vi "RenameMembersSetName.vi"(4 "Output String":string, 6 "Input String":string, 8 "error in (no error)":errorcluster, 10 "Controls":refnum<vi>[](array[refnum]), 11 "LVClassLibrary Refnum":refnum<vi>) -> (0 "error out":errorcluster, 3 "Library Refnum out":refnum<vi>)   [LabVIEW 2014, in "ClassRenamer.lvclass"]
uses:
  ClassRenamer.lvclass
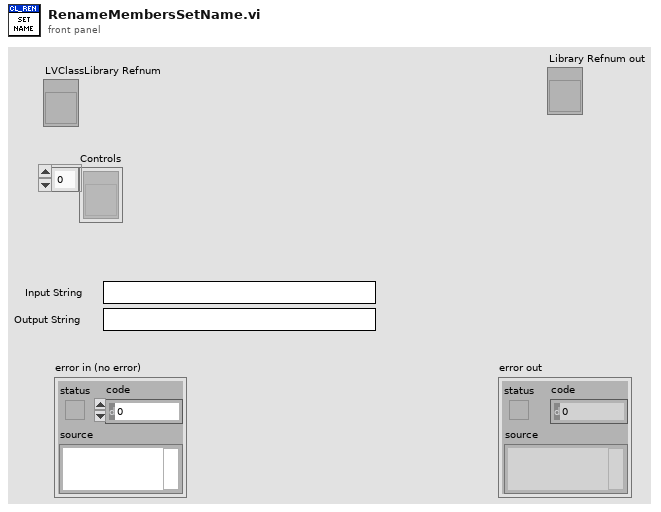
[diagram p1: front panel]
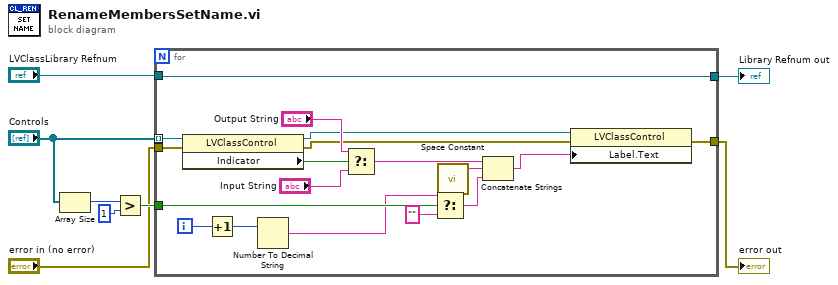
[diagram p0: block diagram]
diagram:
  n1 = Array Size(array="Controls") -> (size(s)=w7:i32)
  n2 = Greater?(x=w7, y=1) -> (0:w4:bool)
  n3 = for {
    tunnel: "Controls" -> [w23] mode=indexing
    tunnel: "LVClassLibrary Refnum" -> [w19]
    tunnel: w4 -> [w16]
    tunnel: [w19] -> w3
    tunnel: "error in (no error)" -> [w18]
    tunnel: [w9] -> w1
    i -> [w26]
    n4 = property class="LVClassControl"(reference=w23, error in=w18) -> (reference out=w10:refnum<vi>, error out=w11:errorcluster, "Indicator"=w22:bool)
    n5 = Increment(x=w26) -> (x+1=w24:i32)
    n6 = Number To Decimal String(number=w24) -> (decimal integer string=w15:string)  [unwired: 1 in]
    n7 = Select(t="Output String", s=w22, f="Input String") -> (s? t:f=w17:string)
    n8 = Select(t=w15, s=w16, f="") -> (s? t:f=w12:string)
    n9 = call <vilib>:"Space Constant.vi"() -> ("String"=w13:string)
    n10 = Concatenate Strings(w17, w13, w12) -> (w25:string)
    n11 = property class="LVClassControl"(reference=w10, error in=w11, "Label.Text"=w25) -> (error out=w9:errorcluster)  [unwired: 1 out]
  }
  "error out" <- w1
  "Library Refnum out" <- w3
